vi "Get configuration chain.vi"(8 "error in (no error)":errorcluster, 11 "TomoBase in":refnum<class "Tomo.lvclass">) -> (0 "error out":errorcluster, 1 "class name":string[](array[string]), 2 "configuration chain":variant[](array[variant]), 3 "TomoBase out":refnum<class "Tomo.lvclass">)   [LabVIEW 2012, in "Tomo.lvclass"]
doc: "Returns an array of variants containing the configuration clusters of each class in the inheritance chain (lowest child class first), together with an array of all class names in the inheritance chain.\n\nFor classes without configuration cluster, the configuration chain contains empty variants."
uses:
  Tomo.lvclass
  <vilib>/Distrio/Murmex/Murmex/Murmex.lvclass
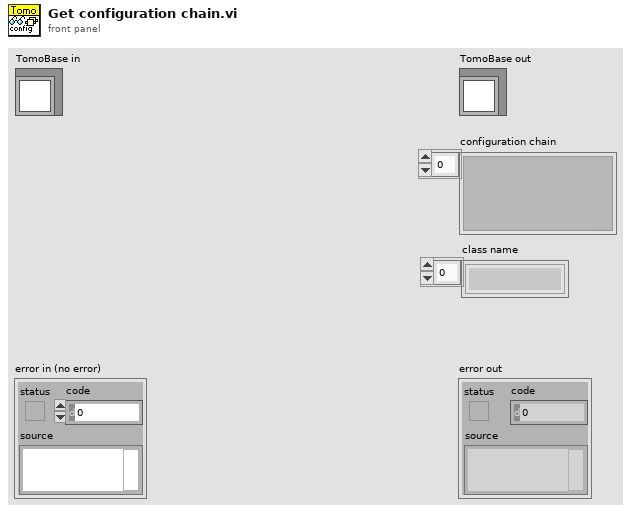
[diagram p1: front panel]
types:
  T1 = typedef "Tomo.lvclass/configuration cluster.ctl" = cluster{"stack component":string, "camera component":string, "stages component":string, "mapping file folder":path, "default stages speed":dbl[unit], "stack overhead time":dbl[unit], "autofocus component":string, "imaging component":string, "AOTF component":string, "pretomo camera x res":u32, "pretomo camera y res":u32, "pretomo full image base path":path, "pretomo small images base path":path, "downsampling factor":u32, "pretomo camera component":string, "pretomo Z step size":dbl[unit], "pretomo X step size":dbl[unit], "pretomo Y step size":dbl[unit], "pretomo camera pixel size":dbl[unit]}
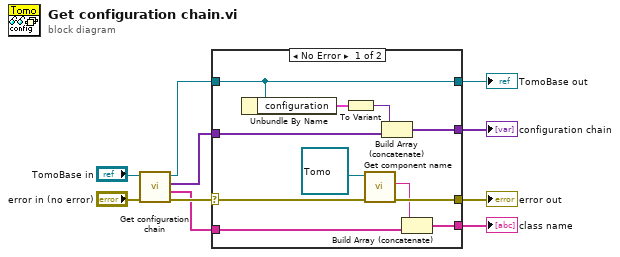
[diagram p0: block diagram]
diagram:
  n1 = call-parent "Get configuration chain.vi"("error in (no error)"="error in (no error)", "MurmexBase in"="TomoBase in") -> ("error out"=w8:errorcluster, "class name"=w6:string[], "configuration chain"=w2:variant[], "MurmexBase out"=w3:refnum<class "Tomo.lvclass">)  [unwired: 6 in]
  n2 = case shown="No Error" w8 {
    selector: w8 -> [w21 w24]
    tunnel: [w19 w24] -> w7
    tunnel: w6 -> [w17 w25]
    tunnel: [w16 w25] -> w5
    tunnel: [w15 w22] -> w4
    tunnel: w3 -> [w15 w22]
    tunnel: w2 -> [w12 w23]
    tunnel: [w11 w23] -> w1
    frame No Error {
      n3 = Unbundle By Name(w15) -> ("configuration"=w14:T1)
      n4 = To Variant(anything=w14) -> (Variant=w13:variant)
      n5 = call <vilib>:"Get component name.vi"("error in (no error)"=w21, "Murmex in"=refnum<class "Tomo.lvclass"> refnum ("Tomo.lvclass")) -> ("error out"=w19:errorcluster, "component name"=w18:string)  [unwired: 7 in, 1 out]
      n6 = Build Array (concatenate)(w13, w12) -> (w11:variant[])
      n7 = Build Array (concatenate)(w18, w17) -> (w16:string[])
    }
    frame Error {
    }
  }
  "error out" <- w7
  "TomoBase out" <- w4
  "configuration chain" <- w1
  "class name" <- w5
